vi "source sep ui.vi"() -> ()   [LabVIEW 2013, in "set source separate.lvclass"]
uses:
  set source separate.lvclass
  <vilib>/CEF_TreeControl/Node/NodeRef.ctl
  <vilib>/CEF_TreeControl/Node/NISE_CEF_Node.lvclass
  <vilib>/NI/AMC/Message Queue.ctl
  <vilib>/NI/AMC/Message.ctl
  <vilib>/NI/Tools/Keyed Array/KeyedArray.ctl
  <vilib>/CEF_TreeControl/Node/UserEventRef.ctl
  <vilib>/CEF_TreeControl/Controls/EventCluster.ctl
  set source separate.lvclass/set source separate.ctl
  Read separate compiled code.vi
  <vilib>/NI/Tools/Keyed Array/Tools_KeyedArray.lvlib
  <vilib>/NI/AMC/AMC.lvlib
  <vilib>/CEF_TreeControl/NISE_CEF_TreeControl.lvlib
panel:
  in  "user event":T1
  in  "main queue":T2
  in  "node ref":T3
  in  "separate compiled code":bool
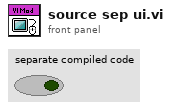
[diagram p1: front panel]
types:
  T1 = typedef "NISE_CEF_Node.lvclass/UserEventRef.ctl" = refnum<user-event>
  T2 = typedef "AMC.lvlib/Message Queue.ctl" = refnum<queue>
  T3 = typedef "NISE_CEF_Node.lvclass/NodeRef.ctl" = refnum<data-value>
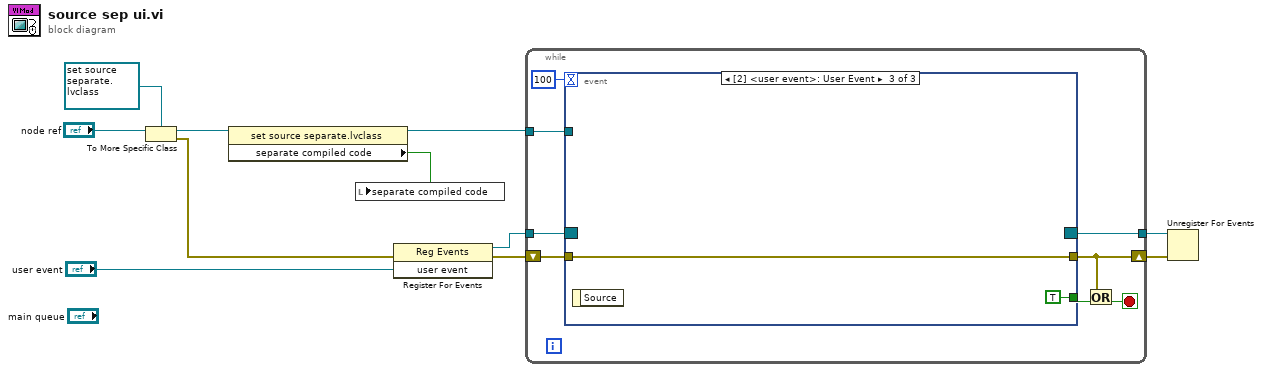
[diagram p0: block diagram]
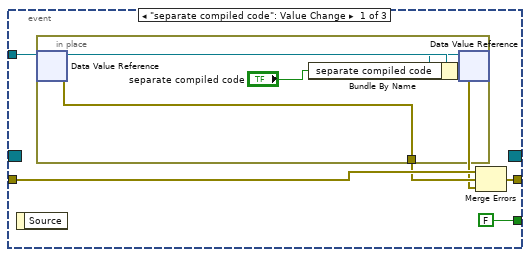
[diagram p2: hidden frame]
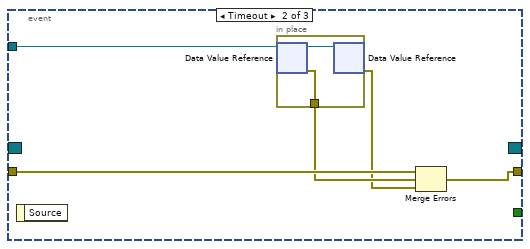
[diagram p3: hidden frame]
diagram:
  n1 = To More Specific Class(target class=refnum<data-value> refnum, reference="node ref") -> (specific class reference=w7:refnum<data-value>, error out=w5:errorcluster)  [unwired: 1 in]
  n2 = property class="set source separate.lvclass"(reference=w7) -> (reference out=w4:refnum<data-value>, "separate compiled code"=w3:bool)  [unwired: 1 in, 1 out]
  n3 = local write "separate compiled code"(w3) -> ()
  n4 = register-events(error in=w5, "user event") -> (reference out=w10:refnum<event-registration>, error out=w11:errorcluster)  [unwired: 1 in]
  n5 = while {
    shift-right: [w12] -> w9
    shift-left: w11 -> [w16]
    tunnel: w10 -> [w19]
    tunnel: [w18] -> w8
    tunnel: w4 -> [w15]
    stop <- w13 stop-if-true
    n6 = event shown="[2] <user event>: User Event" {
      selector: w19 -> [_ _ _]
      dyn-events: [_ _ _] -> w18
      timeout: 100 -> [_ _ _]
      tunnel: [FALSE _ TRUE] -> w17
      tunnel: [w23 w32 w38] -> w12
      tunnel: w16 -> [w25 w33 w38]
      tunnel: w15 -> [w24 w34 _]
      event "separate compiled code": Value Change {
        n7 = event-data() -> ()  [unwired: 1 in, 1 out]
        n8 = in-place {
          in-place-border: [w27] -> w21
          n9 = in-place-dvr #1(w24) -> (w29:refnum<class "set source separate.lvclass">, w27:errorcluster)
          n10 = Bundle By Name(cluster=w29, "separate compiled code"="separate compiled code") -> (w28:refnum<class "set source separate.lvclass">)
          n11 = in-place-dvr #1(w28) -> (w20:errorcluster)  [unwired: 1 out]
        }
        n12 = Merge Errors(w25, w21, w20) -> (w23:errorcluster)
      }
      event Timeout {
        n13 = event-data() -> ()  [unwired: 1 in, 1 out]
        n14 = in-place {
          in-place-border: [w35] -> w31
          n15 = in-place-dvr #2(w34) -> (w36:refnum<class "set source separate.lvclass">, w35:errorcluster)
          n16 = in-place-dvr #2(w36) -> (w30:errorcluster)  [unwired: 1 out]
        }
        n17 = Merge Errors(w33, w31, w30) -> (w32:errorcluster)
      }
      event User Event {
        n18 = event-data() -> ()  [unwired: 1 in, 1 out]
      }
    }
    n19 = Or(x=w12, y=w17) -> (x .or. y?=w13:bool)
  }
  n20 = Unregister For Events(event registration refnum=w8, error in=w9) -> ()  [unwired: 1 out]
